vi "AdjustHeight.vi"(8 "error in (no error)":errorcluster, 10 "VISA resource name":refnum<visa-resource-name>="COM4") -> (0 "error out":errorcluster, 1 "Z Position":dbl, 2 "VISA resource name out":refnum<visa-resource-name>, 3 "controller out":refnum<k24>)   [LabVIEW 2016]
uses:
  C:/Users/TTUHEP/Documents/LabVIEW/Other Models/2010/Bin/Aerotech.A3200.dll
  Other Models/2010/Bin/Aerotech.A3200.dll
  <vilib>/Instr/_visa.llb/VISA Configure Serial Port (Instr).vi
panel:
  in  "baud rate":u32=1500000
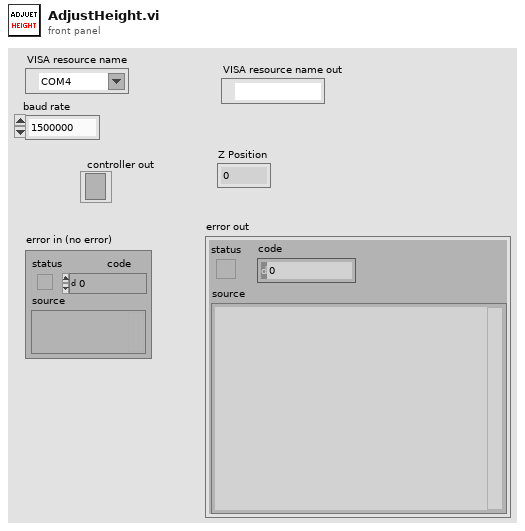
[diagram p1: front panel]
types:
  T1 = typedef "ControllerDiagPacket.ctl" = cluster{"Number of Diag Packets":i32, "Axes":T2[], "error":errorcluster}
  T2 = typedef "AxisDiagPacket.ctl" = cluster{"Axis Name":string, "Analog Input 0":dbl, "Analog Input 1":dbl, "Axis Fault (num)":i32, "Axis Fault (str)":string, "Axis Fault (bits)":cluster{"AmplifierFault":bool, "AmplifierTemperatureFault":bool, "CcwEndOfTravelLimitFault":bool, "CcwSoftwareLimitFault":bool, "CommunicationLostFault":bool, "CwEndOfTravelLimitFault":bool, "CwSoftwareLimitFault":bool, "EmergencyStopFault":bool, "EncoderFault":bool, "ExternalFault":bool, "FeedbackScalingFault":bool, "GantryMisalignFault ":bool, "HallSensorFault":bool, "InPositionTimeoutFault":bool, "InternalFault":bool, "MarkerSearchFault":bool, "MaxVelocityCommandFault":bool, "MissedInterruptFault":bool, "MotorTemperatureFault":bool, "None":bool, "OverCurrentFault":bool, "PositionErrorFault":bool, "PositionFeedbackFault":bool, "PowerSupplyFault":bool, "ProbeInputFault":bool, "SafeZoneFault":bool, "VelocityErrorFault":bool, "VelocityFeedbackFault":bool, "VoltageClampFault":bool}, "Axis Status (num)":i32, "Axis Status (str)":string, "Axis Status (bits)":cluster{"BacklashActive":bool, "CalibrationEnabled1D":bool, "CalibrationEnabled2D":bool, "CommandValid":bool, "DriveAbortPending":bool, "DrivePending":bool, "Enabling":bool, "GainMappingEnabled":bool, "GantryAligned":bool, "GantryRealigning":bool, "Homed":bool, "Homing":bool, "IFOVEnabled":bool, "JogGenerating":bool, "Jogging":bool, "JoystickControl":bool, "MasterSlaveControl":bool, "MotionBlocked":bool, "MotionClamped":bool, "MoveDone":bool, "None":bool, "NotVirtual":bool, "Profiling":bool, "Stability0":bool, "Stability1":bool, "TrajectoryFiltering":bool, "WaitDone":bool}, "Current Command":sgl, "Current Error":sgl, "Current Feedback":sgl, "Digital Inputs":i32, "Digital Outputs":i32, "Drive Status":i32, "Drive Status (str)":string, "Drive Status (bits)":cluster{"AccelerationPhase":bool, "AutofocusActive":bool, "BrakeOutput":bool, "CcwEndOfTravelLimitInput":bool, "CosineEncoderError":bool, "CurrentClamp":bool, "CwEndOfTravelLimitInput":bool, "DecelerationPhase":bool, "DualLoopActive":bool, "EmergencyStopInput":bool, "Enabled":bool, "EncoderClipping":bool, "GalvoCalibrationEnabled":bool, "GalvoPowerCorrection":bool, "HallAInput":bool, "HallBInput":bool, "HallCInput":bool, "HighResolutionMode":bool, "HomeLimitInput":bool, "InPosition":bool, "InPosition2":bool, "MarkerInput":bool, "MarkerLatch":bool, "MoveActive":bool, "NoMotorSupply":bool, "None":bool, "PowerLimiting":bool, "ProgrammingFlash":bool, "ProgrammingMXH":bool, "PSOHaltLatch":bool, "ServoControl":bool, "SineEncoderError":bool}, "Position Feedback Auxiliary":dbl, "Position Command":dbl, "Position Error":dbl, "Position Feedback":dbl, "Program Position Command":dbl, "Program Position Error":dbl, "Program Position Feedback":dbl, "Velocity Command":dbl, "Velocity Error":dbl, "Velocity Feedback":dbl}
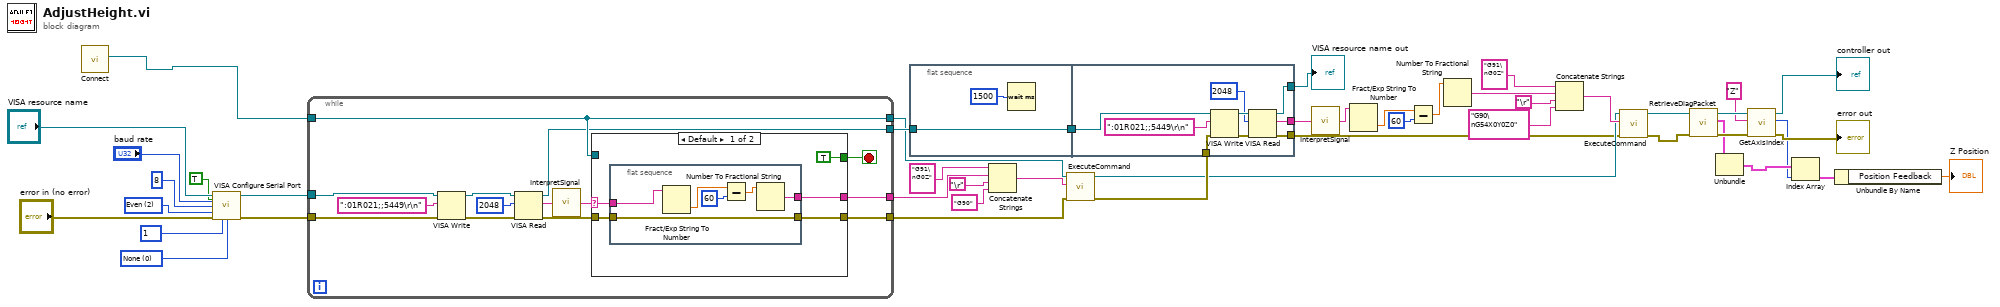
[diagram p0: block diagram]
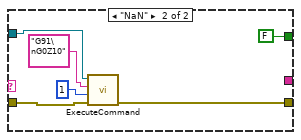
[diagram p2: hidden frame]
diagram:
  w46 = u16 0 items=["None"=0, "XON/XOFF"=1, "RTS/CTS"=2, "DTR/DSR"=4] ("flow control")
  w45 = u16 10 items=["1"=10, "1.5"=15, "2.0"=20] ("stop bits")
  w44 = u16 2 items=["None", "Odd", "Even", "Mark", "Space"] ("parity")
  n1 = call "Connect.vi"() -> ("controller"=w1:refnum<k24>)  [unwired: 10 in, 1 out]
  n2 = call-poly "VISA Configure Serial Port"("VISA resource name"="VISA resource name", "Enable Termination\nChar (T)"=TRUE, "baud rate (9600)"="baud rate", "data bits (8)"=u16 8 ("data bits"), "parity (0:none)"=w44, "error in (no error)"="error in (no error)", "stop bits (10: 1 bit)"=w45, "flow control (0:none)"=w46) -> ("VISA resource name out"=w38:refnum<visa-resource-name>, "error out"=w37:errorcluster)  [unwired: 6 in]
  n3 = while {
    tunnel: w38 -> [w60]
    tunnel: w37 -> [w56]
    tunnel: w1 -> [w50]
    tunnel: [w51] -> w30
    tunnel: [w50] -> w29
    tunnel: [w48] -> w31
    tunnel: [w47] -> w32
    stop <- w49 stop-if-true
    n4 = VISA Write(VISA resource name=w60, write buffer=":01R021;;5449\r\n" ("Command"), error in (no error)=w56) -> (VISA resource name out=w59:refnum<visa-resource-name>, error out=w57:errorcluster)  [unwired: 1 out]
    n5 = VISA Read(VISA resource name=w59, byte count=u32 2048, error in (no error)=w57) -> (VISA resource name out=w47:refnum<visa-resource-name>, read buffer=w54:string, error out=w52:errorcluster)  [unwired: 1 out]
    n6 = call "InterpretSignal.vi"("String in"=w54) -> ("String out"=w53:string)
    n7 = case shown="Default" w53 {
      selector: w53 -> [w62 _]
      tunnel: w50 -> [_ w77]
      tunnel: w52 -> [w61 w74]
      tunnel: [w63 w73] -> w51
      tunnel: [TRUE FALSE] -> w49
      tunnel: [w64 _] -> w48
      frame Default {
        n8 = flat-sequence {
          tunnel: [w68] -> w64
          tunnel: [w66] -> w63
          tunnel: w62 -> [w67]
          tunnel: w61 -> [w66]
          frame #0 {
            n9 = Fract/Exp String To Number(string=w67) -> (number=w71:dbl)  [unwired: 3 in, 1 out]
            n10 = Subtract(x=w71, y=60) -> (x-y=w69:dbl)
            n11 = Number To Fractional String(number=w69) -> (F-format string=w68:string)  [unwired: 3 in]
          }
        }
      }
      frame "NaN" {
        n12 = call "ExecuteCommand.vi"("error in (no error)"=w74, "taskId"=1, "Command Code"="G91\nG0Z10", "controller in"=w77) -> ("error out"=w73:errorcluster)  [unwired: 5 in, 2 out]
      }
    }
  }
  n13 = flat-sequence {
    tunnel: w32 -> [w79]
    tunnel: [w79] -> w17
    tunnel: w28 -> [w84]
    tunnel: [w82] -> w27
    tunnel: [w81] -> w18
    tunnel: w17 -> [w88]
    tunnel: [w80] -> w14
    frame #0 {
      n14 = Wait (ms)(milliseconds to wait=1500) -> ()  [unwired: 1 out]
    }
    frame #1 {
      n15 = VISA Write(VISA resource name=w88, write buffer=":01R021;;5449\r\n" ("Command"), error in (no error)=w84) -> (VISA resource name out=w87:refnum<visa-resource-name>, error out=w83:errorcluster)  [unwired: 1 out]
      n16 = VISA Read(VISA resource name=w87, byte count=u32 2048, error in (no error)=w83) -> (VISA resource name out=w80:refnum<visa-resource-name>, read buffer=w82:string, error out=w81:errorcluster)  [unwired: 1 out]
    }
  }
  n17 = Concatenate Strings("G91\nG0Z", w31, "\r", "G90") -> (w35:string)
  n18 = call "ExecuteCommand.vi"("error in (no error)"=w30, "Command Code"=w35, "controller in"=w29) -> ("error out"=w28:errorcluster, "controller out"=w19:refnum<k24>)  [unwired: 6 in, 1 out]
  n19 = call "InterpretSignal.vi"("String in"=w27) -> ("String out"=w24:string)
  n20 = Fract/Exp String To Number(string=w24) -> (number=w23:dbl)  [unwired: 3 in, 1 out]
  n21 = Subtract(x=w23, y=60) -> (x-y=w21:dbl)
  n22 = Number To Fractional String(number=w21) -> (F-format string=w20:string)  [unwired: 3 in]
  n23 = Concatenate Strings("G91\nG0Z", w20, "\r", "G90\nG54X0Y0Z0") -> (w25:string)
  n24 = call "ExecuteCommand.vi"("error in (no error)"=w18, "Command Code"=w25, "controller in"=w19) -> ("error out"=w12:errorcluster, "controller out"=w13:refnum<k24>)  [unwired: 6 in, 1 out]
  n25 = call "RetrieveDiagPacket.vi"("error in (no error)"=w12, "Controller In"=w13) -> ("error out"=w10:errorcluster, "ControllerDiagPacket"=w6:T1, "Controller Out"=w11:refnum<k24>)  [unwired: 7 in]
  n26 = Unbundle(w6) -> ("Axes"=w5:T2[])  [unwired: 2 out]
  n27 = call "GetAxisIndex.vi"("error in (no error)"=w10, "axis name"="Z", "controller in"=w11) -> ("error out"=→"error out":errorcluster, "axis index"=w4:i32, "controller out"=→"controller out":refnum<k24>)  [unwired: 6 in]
  n28 = Index Array(array=w5, index=w4) -> (element=w3:T2)
  n29 = Unbundle By Name(w3) -> ("Position Feedback"=→"Z Position":dbl)
  "VISA resource name out" <- w14
